vi "ModBUS Test.vi"() -> ()   [LabVIEW 2023]
uses:
  <vilib>/NI/Modbus Library/API/Master/Modbus Master.lvclass
  PIDModBus/PIDModbus.lvlib
panel:
  out "error out":errorcluster
  out "Temperature (C)":dbl
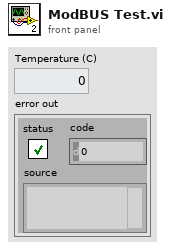
[diagram p1: front panel]
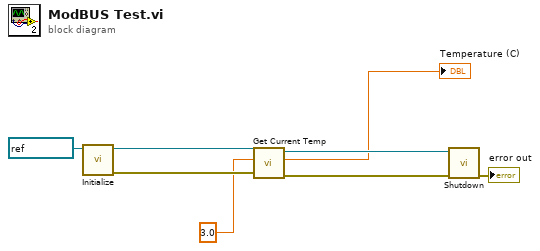
[diagram p0: block diagram]
diagram:
  n1 = call "Initialize.vi"("VISA resource name"=refnum<visa-resource-name> "COM5") -> ("error out"=w6:errorcluster, "session out"=w7:refnum<class "Modbus Master.lvclass">)  [unwired: 9 in]
  n2 = call "Get Current Temp.vi"("error in (no error)"=w6, "TempSP"=3.0, "Modbus Master in"=w7) -> ("error out"=w3:errorcluster, "Temperature (C)"=→"Temperature (C)":dbl, "Modbus Master out"=w4:refnum<class "Modbus Master.lvclass">)  [unwired: 5 in, 1 out]
  n3 = call-dynamic "Shutdown.vi"("error in"=w3, "Modbus master in"=w4) -> ("error out"=→"error out":errorcluster)  [unwired: 9 in]
